vi "Test_BufferedLogBufferFull_EventsCaptured.vi"(8 "error in (no error)":errorcluster, 11 "TestCase in":refnum<class "TestBufferedLogSink.lvclass">) -> (0 "error out":errorcluster, 3 "TestCase out":refnum<class "TestBufferedLogSink.lvclass">)   [LabVIEW 2019, in "TestBufferedLogSink.lvclass"]
uses:
  TestBufferedLogSink.lvclass
  Source/Composed Log/LoggerReference/LoggerReference.lvclass/LoggerReference.ctl
  Source/LVQueue Sink/LVQueue Sink.lvclass/LVQueue Sink.ctl
  b83ac39a-525a-4956-83d8-1e446c51aff0.vi
  Source/Composed Log/LoggerReference/Return Aggregate Queues.vi
  Source/Composed Log/LoggerReference/Add Aggregate Log.vi
  b83ac39a-525a-4956-83d8-1e446c51aff0.vi/09091709-1b71-4528-a91a-0c4137ae06fc.vi
  Source/Composed Log/LoggerReference/Log.vi
  Source/Composed Log/LoggerReference/Get Valid Event Time.vi
  Source/Composed Log/LoggerReference/Send Add Sink.vi
  Source/Composed Log/LoggerReference/Remove Stale Logs.vi
  Source/LVQueue Sink/LVQueue Sink.lvclass
  C:/CS/Log/Source/Composed Log/Log Sink/Log Sink.lvclass
  Source/Buffered Log Sink/Buffered Log Sink.lvclass
  Source/Composed Log/Application Logger/Launch Worker Loop.vi
  Source/Composed Log/LoggerReference/Initialize Logger Instance.vi
  Source/Composed Log/LoggerReference/LoggerReference.lvclass
  Source/Composed Log/IErrorFormat/IErrorFormat.lvclass
  Source/Composed Log/Log Sink/Log Sink.lvclass
  <vilib>/addons/_JKI Toolkits/VI Tester/TestCase.llb/TestCase.lvclass
  C:/Program Files (x86)/National Instruments/LabVIEW 2019/vi.lib/addons/_JKI Toolkits/VI Tester/TestCase.llb/TestCase.lvclass
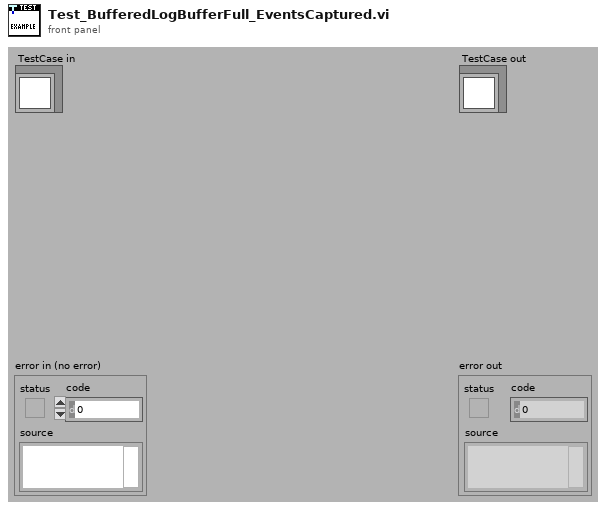
[diagram p1: front panel]
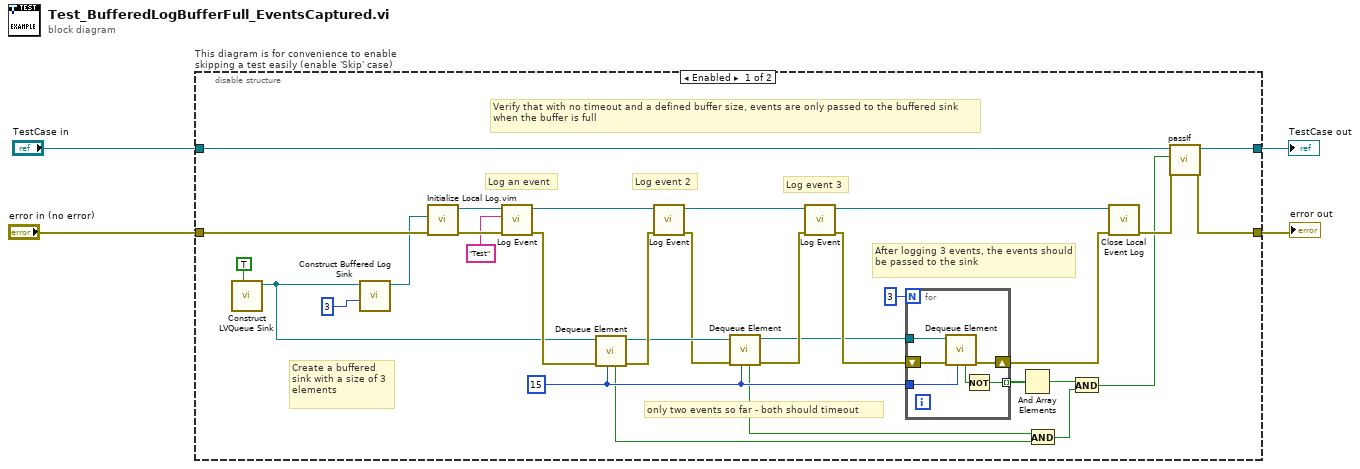
[diagram p0: block diagram]
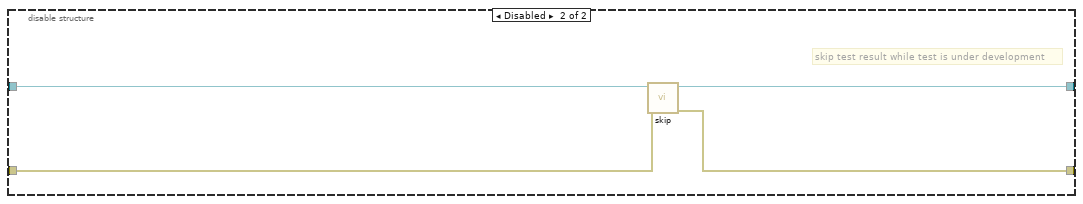
[diagram p2: hidden frame]
diagram:
  n1 = disable-structure "This diagram is for convenience to enable skipping a test easily (enable 'Skip' case)" shown="Enabled" {
    disable-tunnel: "TestCase in" -> [w29 w45]
    disable-tunnel: [w28 w43] -> w1
    disable-tunnel: [w27 w44] -> w3
    disable-tunnel: "error in (no error)" -> [w25 w42]
    frame Enabled {
      w13 = 15 ("timeout in ms (-1)")
      # "Verify that with no timeout and a defined buffer size, events are only passed to the buffered sink when the buffer is full"
      # "Log event 3"
      # "Log event 2"
      # "After logging 3 events, the events should be passed to the sink"
      # "only two events so far - both should timeout"
      # "Log an event"
      # "Create a buffered sink with a size of 3 elements"
      n2 = call "Construct LVQueue Sink.vi"("User Shutdown? (F)"=TRUE) -> ("LVQueue Sink out"=w31:refnum<class "LVQueue Sink.lvclass">)  [unwired: 9 in, 1 out]
      n3 = call "Construct Buffered Log Sink.vi"("Buffer Size (128)"=3 ("Buffer Timeout ms (-1)"), "Sink to Buffer"=w31) -> ("Buffered Log Sink out"=w5:refnum<class "Buffered Log Sink.lvclass">)  [unwired: 9 in]
      n4 = call "Initialize Local Log.vim"("error in (no error)"=w25, "Startup Sink(s)"=w5) -> ("error out"=w35:errorcluster, "Log Instance Reference"=w34:refnum<class "LoggerReference.lvclass">)  [unwired: 7 in, 1 out]
      n5 = call "Log Event.vi"("error in (no error)"=w35, "SourceID"="Test", "Log Instance"=w34) -> ("error out"=w32:errorcluster, "Log Instance Out"=w23:refnum<class "LoggerReference.lvclass">)  [unwired: 7 in]
      n6 = call "Dequeue Element.vi"("timeout in ms (-1)"=w13, "error in (no error)"=w32, "LVQueue Sink in"=w31) -> ("error out"=w20:errorcluster, "LVQueue Sink out"=w19:refnum<class "LVQueue Sink.lvclass">, "Timed Out?"=w10:bool)  [unwired: 5 in, 1 out]
      n7 = call "Log Event.vi"("error in (no error)"=w20, "Log Instance"=w23) -> ("error out"=w18:errorcluster, "Log Instance Out"=w22:refnum<class "LoggerReference.lvclass">)  [unwired: 8 in]
      n8 = call "Dequeue Element.vi"("timeout in ms (-1)"=w13, "error in (no error)"=w18, "LVQueue Sink in"=w19) -> ("error out"=w17:errorcluster, "LVQueue Sink out"=w15:refnum<class "LVQueue Sink.lvclass">, "Timed Out?"=w11:bool)  [unwired: 5 in, 1 out]
      n9 = call "Log Event.vi"("error in (no error)"=w17, "Log Instance"=w22) -> ("error out"=w16:errorcluster, "Log Instance Out"=w21:refnum<class "LoggerReference.lvclass">)  [unwired: 8 in]
      n10 = for {
        N: 3 -> [_]
        tunnel: w15 -> [w40]
        tunnel: w13 -> [w39]
        tunnel: [w36] -> w9 mode=indexing
        shift-right: [w37] -> w12
        shift-left: w16 -> [w41]
        n11 = call "Dequeue Element.vi"("timeout in ms (-1)"=w39, "error in (no error)"=w41, "LVQueue Sink in"=w40) -> ("error out"=w37:errorcluster, "Timed Out?"=w38:bool)  [unwired: 5 in, 2 out]
        n12 = Not(x=w38) -> (.not. x?=w36:bool)
      }
      n13 = And Array Elements(Boolean array=w9) -> (logical AND=w8:bool)
      n14 = And(x=w11, y=w10) -> (x .and. y?=w7:bool)
      n15 = And(x=w8, y=w7) -> (x .and. y?=w6:bool)
      n16 = call "Close Local Event Log.vi"("error in (no error)"=w12, "Log Instance"=w21) -> ("error out"=w26:errorcluster)  [unwired: 9 in]
      n17 = call-dynamic "passIf.vi"("error in (no error)"=w26, "pass"=w6, "TestCase in"=w29) -> ("error out"=w27:errorcluster, "TestCase out"=w28:refnum<class "TestBufferedLogSink.lvclass">)  [unwired: 7 in]
    }
    frame Disabled {
      # "skip test result while test is under development"
      n18 = call <vilib>:"skip.vi"("error in (no error)"=w42, "TestCase in"=w45) -> ("error out"=w44:errorcluster, "TestCase out"=w43:refnum<class "TestBufferedLogSink.lvclass">)  [unwired: 8 in]
    }
  }
  "error out" <- w3
  "TestCase out" <- w1
